vi "Dispersive_Stress.vi"() -> (0 "New Values In":string[][](array[string])=[["Test data5"]], 1 "New Chs In":string[](array[string])=["30-10-03:New:Channel new5"])   [LabVIEW 2021]
uses:
  Results_plotter_Global.vi
  <vilib>/Analysis/NI_AALBase.lvlib
  <vilib>/Analysis/baseanly.llb/Mean (DBL).vi
  Data plotting/subVIs/Plot_Values_Global.vi
  Controls/ok_button.ctl
panel:
  in  "Cancel Button":bool
  out "Message":string
  in  "OK":T1
  in  "Product Name":string="uw/Ur^2:Disp"
  in  "Second Dispersive Name":string="w^2/Ur^2:Disp"
  in  "First Dispersive Name":string="u^2/Ur^2:Disp"
  out "Second Variable":string
  out "First Variable":string
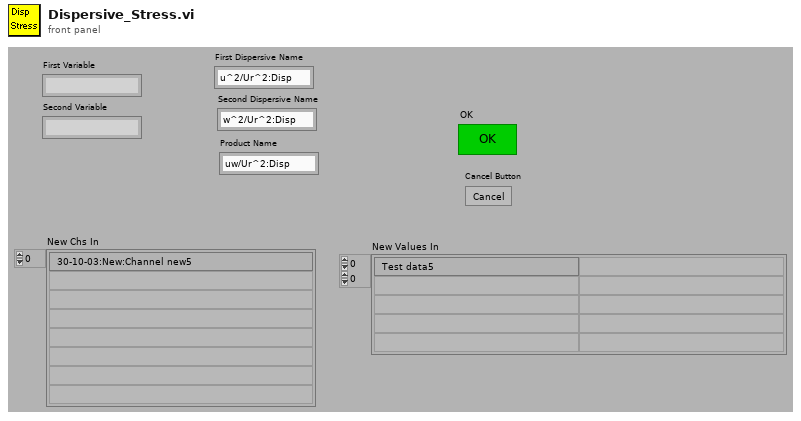
[diagram p1: front panel]
types:
  T1 = typedef "ok_button.ctl" = bool
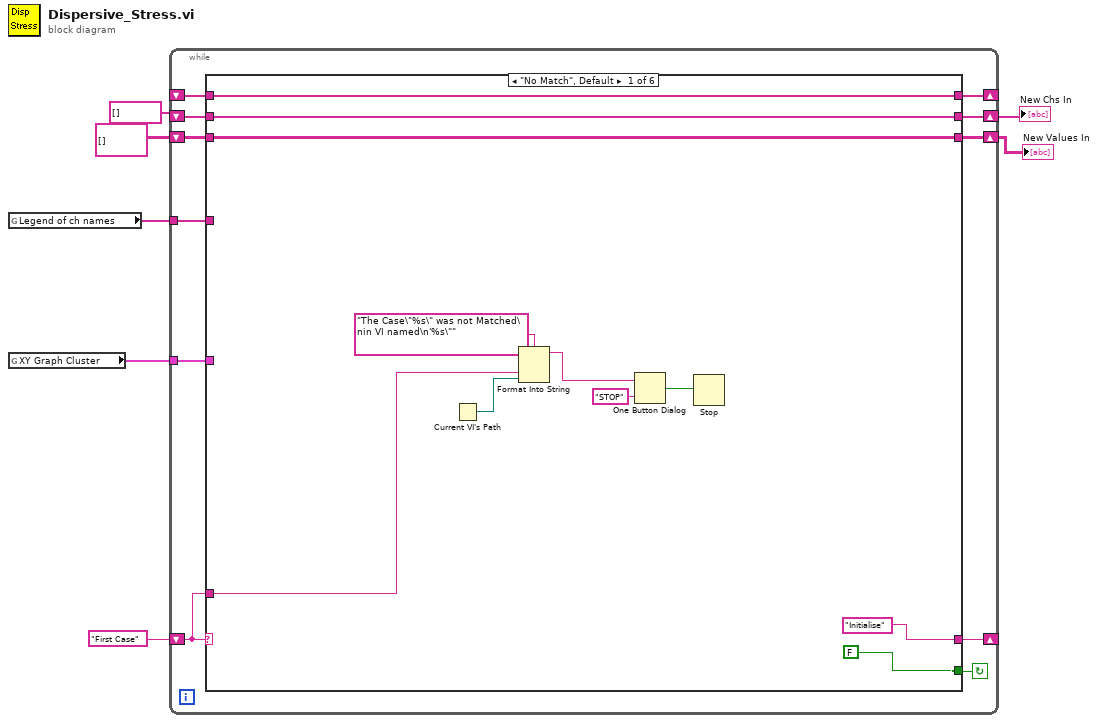
[diagram p0: block diagram]
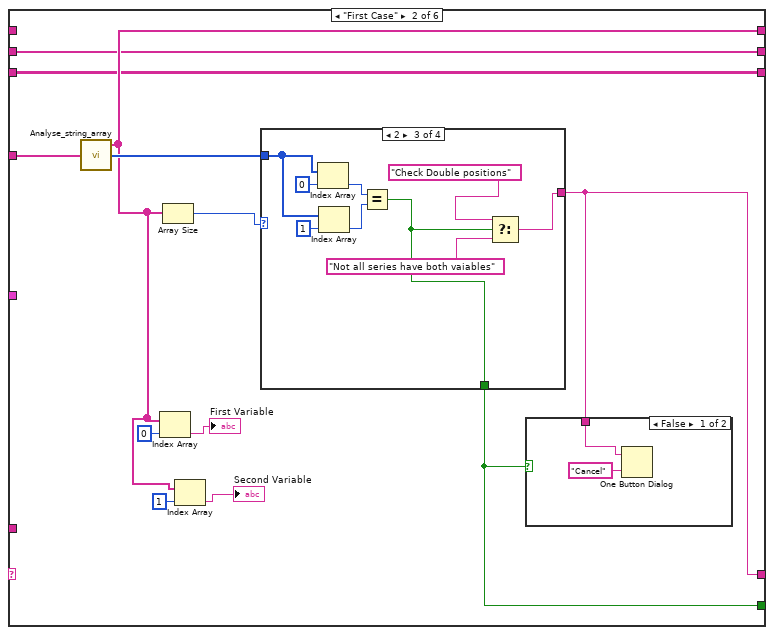
[diagram p2: hidden frame]
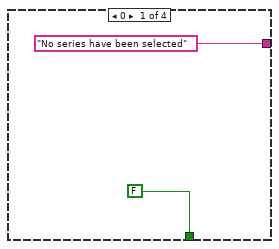
[diagram p4: hidden frame]
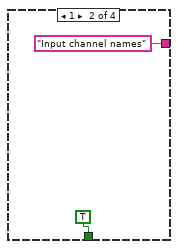
[diagram p5: hidden frame]
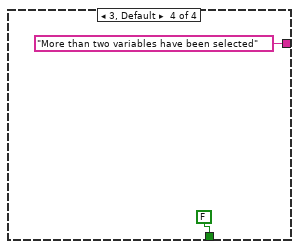
[diagram p6: hidden frame]
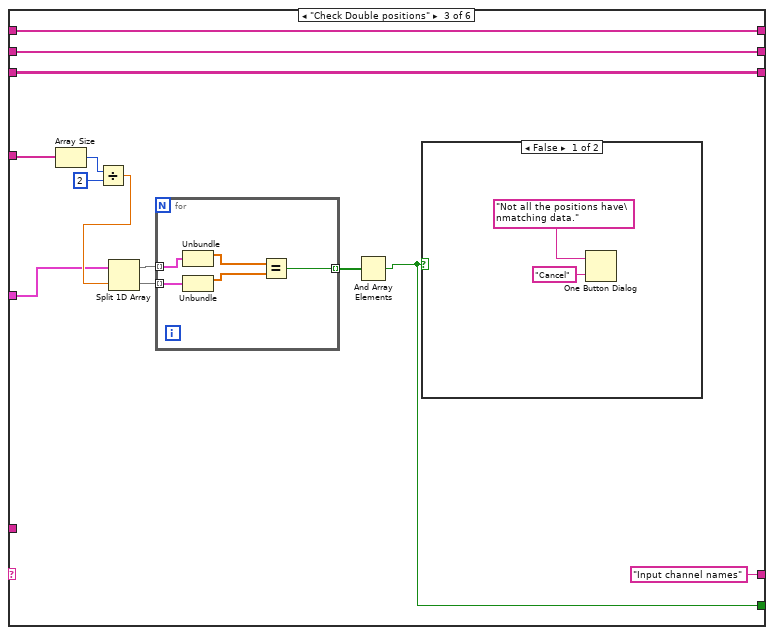
[diagram p7: hidden frame]
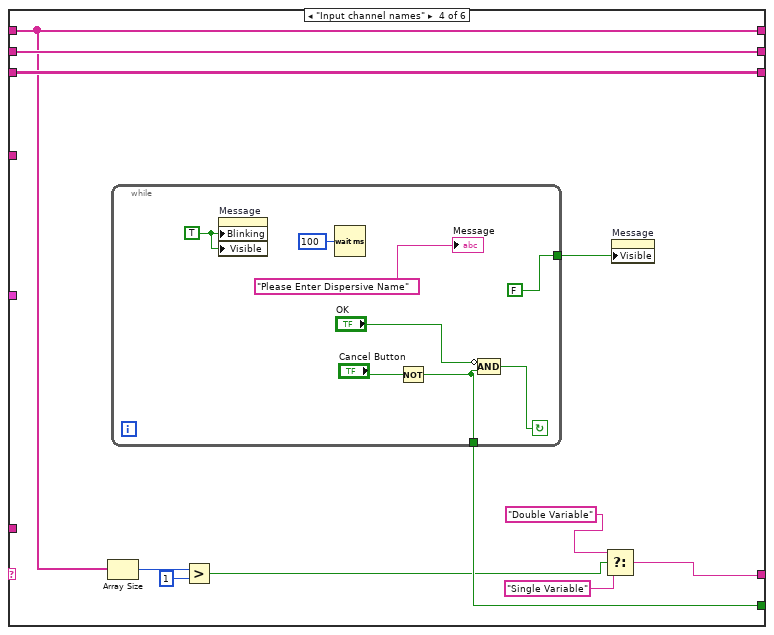
[diagram p9: hidden frame]
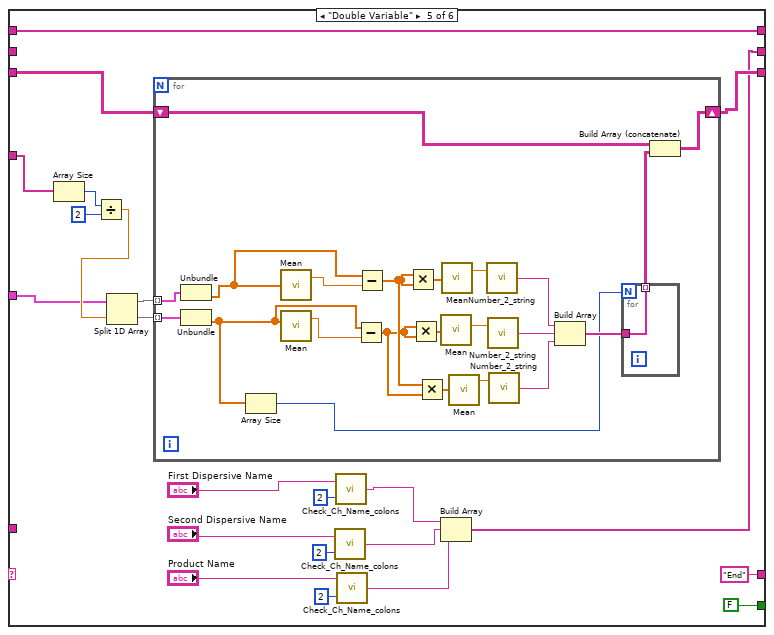
[diagram p10: hidden frame]
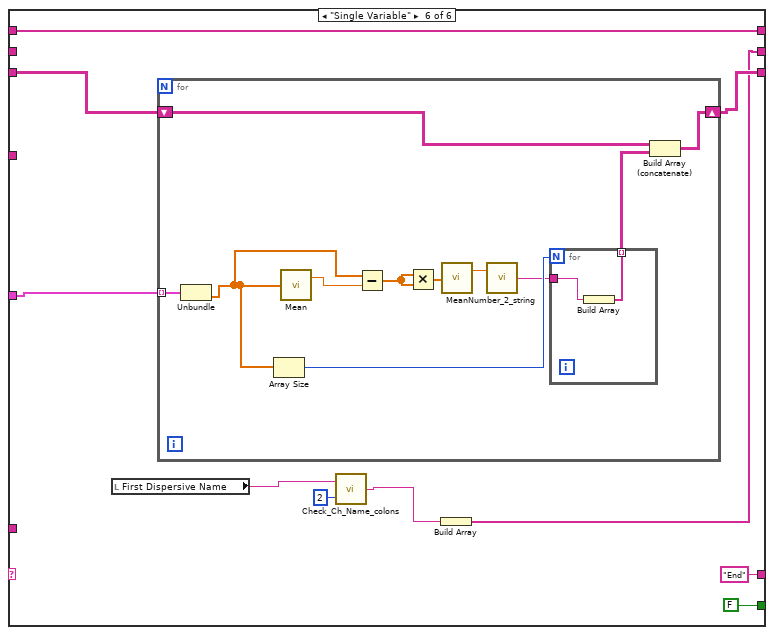
[diagram p11: hidden frame]
diagram:
  n1 = global read "Results_plotter_Global.vi" "Legend of ch names"() -> (w6:string[])
  n2 = global read "Plot_Values_Global.vi" "XY Graph Cluster"() -> (w1:cluster{dbl[], dbl[]}[])
  n3 = while {
    shift-left: "First Case" -> [w16]
    shift-right: [w17] -> _
    tunnel: w6 -> [w15]
    shift-right: [w14] -> _
    shift-left: _ -> [w13]
    tunnel: w1 -> [w12]
    shift-right: [w11] -> w4
    shift-left: string[][] [] -> [w10]
    shift-right: [w9] -> w3
    shift-left: string[] [] -> [w8]
    stop <- w18 continue-if-true
    n4 = case shown="\"No Match\", Default" w16 {
      tunnel: [FALSE w39 w63 w85 FALSE FALSE] -> w18
      tunnel: ["Initialise" w38 "Input channel names" ("f") w81 "End" ("f") "End" ("f")] -> w17
      tunnel: w16 -> [w24 _ _ _ _ _]
      tunnel: w15 -> [_ w41 w71 _ w111 _]
      tunnel: [w21 w34 w60 w87 w112 w151] -> w14
      tunnel: w13 -> [w21 _ w60 w87 w112 w151]
      tunnel: w12 -> [_ _ w67 _ w116 w145]
      tunnel: [w19 w30 w61 w89 w113 w152] -> w11
      tunnel: w10 -> [w19 w30 w61 w89 w109 w143]
      tunnel: [w20 w31 w59 w88 w99 w147] -> w9
      tunnel: w8 -> [w20 w31 w59 w88 _ _]
      frame "No Match", Default {
        n5 = Current VI's Path() -> (path=w23:path)
        n6 = Format Into String(format string="The Case\"%s\" was not Matched\nin VI named\n'%s\"" ("Format String"), w24, w23) -> (resulting string=w27:string)  [unwired: 2 in, 1 out]
        n7 = One Button Dialog(message=w27, button name ("OK")="STOP") -> (true=w25:bool)
        n8 = Stop(stop? (T)=w25) -> ()
      }
      frame "First Case" {
        n9 = call "Analyse_string_array.vi"("String array"=w41) -> ("Unique strings"=w34:string[], "Frequency"=w37:i32[])  [unwired: 1 in]
        n10 = Index Array(array=w34, index=0) -> (element=→"First Variable":string)
        n11 = Array Size(array=w34) -> (size(s)=w40:i32)
        n12 = Index Array(array=w34, index=1) -> (element=→"Second Variable":string)
        n13 = case shown="2" w40 {
          tunnel: [FALSE TRUE w51 FALSE] -> w39
          tunnel: ["No series have been selected" "Input channel names" w49 "More than two variables have been selected"] -> w38
          tunnel: w37 -> [_ _ w54 _]
          frame 0 {
          }
          frame 1 {
          }
          frame 2 {
            n14 = Index Array(array=w54, index=0) -> (element=w52:i32)
            n15 = Index Array(array=w54, index=1) -> (element=w53:i32)
            n16 = Equal?(x=w52, y=w53) -> (x = y?=w51:bool)
            n17 = Select(t="Check Double positions", s=w51, f="Not all series have both vaiables") -> (s? t:f=w49:string)
          }
          frame 3, Default {
          }
        }
        n18 = case shown="False" w39 {
          tunnel: w38 -> [w43 _]
          frame False {
            n19 = One Button Dialog(message=w43, button name ("OK")="Cancel") -> ()  [unwired: 1 out]
          }
          frame True {
          }
        }
      }
      frame "Check Double positions" {
        n20 = Array Size(array=w71) -> (size(s)=w70:i32)
        n21 = Divide(x=w70, y=2) -> (x/y=w68:dbl)
        n22 = Split 1D Array(array=w67, index=w68) -> (first subarray=w66:cluster{dbl[], dbl[]}[], second subarray=w65:cluster{dbl[], dbl[]}[])
        n23 = for {
          tunnel: w66 -> [w78] mode=indexing
          tunnel: w65 -> [w77] mode=indexing
          tunnel: [w74] -> w64 mode=indexing
          n24 = Unbundle(w78) -> (w76:dbl[])  [unwired: 1 out]
          n25 = Unbundle(w77) -> (w75:dbl[])  [unwired: 1 out]
          n26 = Equal?(x=w76, y=w75) -> (x = y?=w74:bool)
        }
        n27 = And Array Elements(Boolean array=w64) -> (logical AND=w63:bool)
        n28 = case shown="False" w63 {
          frame False {
            n29 = One Button Dialog(message="Not all the positions have\nmatching data.", button name ("OK")="Cancel") -> ()  [unwired: 1 out]
          }
          frame True {
          }
        }
      }
      frame "Input channel names" {
        n30 = Array Size(array=w87) -> (size(s)=w84:i32)
        n31 = while {
          tunnel: [FALSE] -> w86
          tunnel: [w90] -> w85
          stop <- w91 continue-if-true
          w94 = TRUE ("Blinking")
          n32 = property on="Message" class="Str"("Blinking"=w94, "Visible"=w94) -> ()  [unwired: 2 in, 2 out]
          n33 = Wait (ms)(milliseconds to wait=u32 100) -> ()  [unwired: 1 out]
          n34 = Not(x="Cancel Button") -> (.not. x?=w90:bool)
          n35 = Compound Arithmetic op=AND(invert "OK", w90) -> (w91:T1)
          "Message" <- "Please Enter Dispersive Name" ("Message")
        }
        n36 = Greater?(x=w84, y=1) -> (0:w82:bool)
        n37 = Select(t="Double Variable", s=w82, f="Single Variable") -> (s? t:f=w81:string)
        n38 = property on="Message" class="Str"("Visible"=w86) -> ()  [unwired: 2 in, 2 out]
      }
      frame "Double Variable" {
        n39 = Array Size(array=w111) -> (size(s)=w119:i32)
        n40 = Divide(x=w119, y=2) -> (x/y=w117:dbl)
        n41 = Split 1D Array(array=w116, index=w117) -> (first subarray=w115:cluster{dbl[], dbl[]}[], second subarray=w114:cluster{dbl[], dbl[]}[])
        n42 = for {
          tunnel: w115 -> [w141] mode=indexing
          tunnel: w114 -> [w140] mode=indexing
          shift-right: [w120] -> w113
          shift-left: w109 -> [w121]
          n43 = Unbundle(w141) -> (w138:dbl[])  [unwired: 1 out]
          n44 = Unbundle(w140) -> (w136:dbl[])  [unwired: 1 out]
          n45 = Array Size(array=w136) -> (size(s)=w133:i32)
          n46 = call-poly <vilib>:"Mean.vi"("X"=w138) -> ("mean"=w139:dbl)  [unwired: 1 out]
          n47 = call-poly <vilib>:"Mean.vi"("X"=w136) -> ("mean"=w137:dbl)  [unwired: 1 out]
          n48 = Subtract(x=w136, y=w137) -> (x-y=w129:dbl[])
          n49 = Subtract(x=w138, y=w139) -> (x-y=w130:dbl[])
          n50 = Multiply(x=w130, y=w130) -> (x*y=w132:dbl[])
          n51 = Multiply(x=w129, y=w129) -> (x*y=w131:dbl[])
          n52 = Multiply(x=w130, y=w129) -> (x*y=w128:dbl[])
          n53 = call-poly <vilib>:"Mean.vi"("X"=w131) -> ("mean"=w127:dbl)  [unwired: 1 out]
          n54 = call-poly <vilib>:"Mean.vi"("X"=w132) -> ("mean"=w126:dbl)  [unwired: 1 out]
          n55 = call-poly <vilib>:"Mean.vi"("X"=w128) -> ("mean"=w125:dbl)  [unwired: 1 out]
          n56 = call "Number_2_string.vi"("number"=w126) -> ("String"=w124:string)  [unwired: 1 in]
          n57 = call "Number_2_string.vi"("number"=w127) -> ("String"=w123:string)  [unwired: 1 in]
          n58 = call "Number_2_string.vi"("number"=w125) -> ("String"=w122:string)  [unwired: 1 in]
          n59 = Build Array(w124, w123, w122) -> (w134:string[])
          n60 = for {
            N: w133 -> [_]
            tunnel: [w142] -> w135 mode=indexing
            tunnel: w134 -> [w142]
          }
          n61 = Build Array (concatenate)(w121, w135) -> (w120:string[][])
        }
        n62 = call "Check_Ch_Name_colons.vi"("No of Colons"=2, "Ch Name in"="Second Dispersive Name") -> ("Ch Name out"=w101:string)
        n63 = call "Check_Ch_Name_colons.vi"("No of Colons"=2, "Ch Name in"="First Dispersive Name") -> ("Ch Name out"=w102:string)
        n64 = call "Check_Ch_Name_colons.vi"("No of Colons"=2, "Ch Name in"="Product Name") -> ("Ch Name out"=w100:string)
        n65 = Build Array(w102, w101, w100) -> (w99:string[])
      }
      frame "Single Variable" {
        n66 = local read "First Dispersive Name"() -> (w144:string)
        n67 = for {
          shift-right: [w158] -> w152
          shift-left: w143 -> [w159]
          tunnel: w145 -> [w157] mode=indexing
          n68 = Unbundle(w157) -> (w156:dbl[])  [unwired: 1 out]
          n69 = Array Size(array=w156) -> (size(s)=w155:i32)
          n70 = call-poly <vilib>:"Mean.vi"("X"=w156) -> ("mean"=w163:dbl)  [unwired: 1 out]
          n71 = Subtract(x=w156, y=w163) -> (x-y=w161:dbl[])
          n72 = Multiply(x=w161, y=w161) -> (x*y=w162:dbl[])
          n73 = call-poly <vilib>:"Mean.vi"("X"=w162) -> ("mean"=w160:dbl)  [unwired: 1 out]
          n74 = call "Number_2_string.vi"("number"=w160) -> ("String"=w154:string)  [unwired: 1 in]
          n75 = for {
            N: w155 -> [_]
            tunnel: w154 -> [w165]
            tunnel: [w164] -> w153 mode=indexing
            n76 = Build Array(w165) -> (w164:string[])
          }
          n77 = Build Array (concatenate)(w159, w153) -> (w158:string[][])
        }
        n78 = call "Check_Ch_Name_colons.vi"("No of Colons"=2, "Ch Name in"=w144) -> ("Ch Name out"=w148:string)
        n79 = Build Array(w148) -> (w147:string[])
      }
    }
  }
  "New Chs In" <- w3
  "New Values In" <- w4
